vi "4stringConc.vi"(1 "ADC bytes":u8[](array[numeric]) format="%x") -> (0 "number hexa":u32)   [LabVIEW 2020]
panel:
  out "concatenated string":string
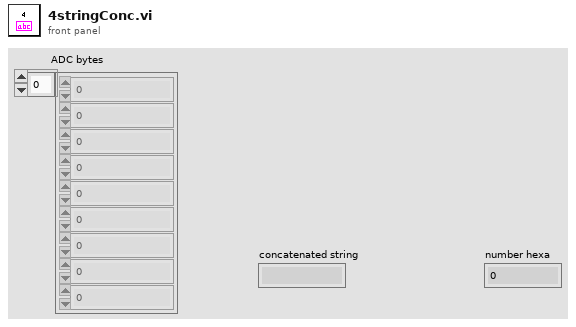
[diagram p1: front panel]
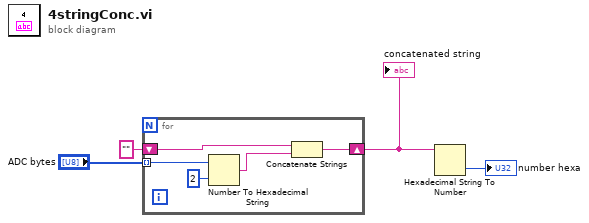
[diagram p0: block diagram]
diagram:
  n1 = for {
    tunnel: "ADC bytes" -> [w8] mode=indexing
    shift-right: [w9] -> w4
    shift-left: "" -> [w6]
    n2 = Number To Hexadecimal String(1:i16 2 ("width (-)"), 2:w8) -> (0:w7:string)
    n3 = Concatenate Strings(w6, w7) -> (w9:string)
  }
  "concatenated string" <- w4
  n4 = Hexadecimal String To Number(string=w4) -> (number=→"number hexa":u32)  [unwired: 2 in, 1 out]
